vi "locationsToWL.vi"(10 "Locations index":dbl[](array[numeric]), 11 "WL Values":dbl[](array[numeric])) -> (3 "Locations WL":dbl[](array[numeric]))   [LabVIEW 2021]
doc: "Random Laser Project\nAndré Romero - 2020\nandretec@ifsc.usp.br\n\nConvert index Locations to Wavelenght"
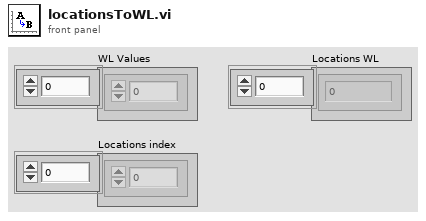
[diagram p1: front panel]
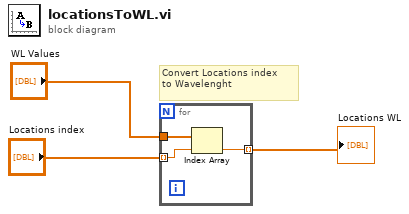
[diagram p0: block diagram]
diagram:
  # "Convert Locations index \nto Wavelenght"
  n1 = for {
    tunnel: "WL Values" -> [w6]
    tunnel: "Locations index" -> [w5] mode=indexing
    tunnel: [w4] -> w3 mode=indexing
    n2 = Index Array(array=w6, index=w5) -> (element=w4:dbl)
  }
  "Locations WL" <- w3
